vi "Target aquisition.vi"(8 "Ring Light Color":T2={"Hue"={119.53551591960586, 182.50767725024022}, "Sat"={103.21428571428572, 255.0}, "Val"={133.57142857142858, 255.0}} {"Hue" scale=0.0..255.0 scale format="%#_3g"}, 11 "Image":T3) -> (0 "Target tracking data":T1, 3 "Threshold image":T3, 4 "is there a target":bool)   [LabVIEW 2014]
uses:
  <vilib>/vision/Image Controls.llb/IMAQ Image.ctl
  <vilib>/vision/NI_Vision_Development_Module.lvlib
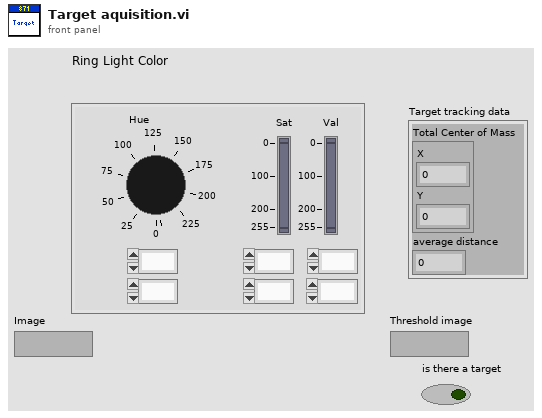
[diagram p1: front panel]
types:
  T1 = cluster{"Total Center of Mass":cluster{"X":dbl, "Y":dbl}, "average distance":dbl}
  T2 = cluster{"Hue":cluster{dbl, dbl}, "Sat":cluster{dbl, dbl}, "Val":cluster{dbl, dbl}}
  T3 = typedef "IMAQ Image.ctl" = refnum<image>
  T4 = cluster{"Area":dbl, "Number of Holes":dbl, "Bounding Rect":cluster{"Left":dbl, "Top":dbl, "Right":dbl, "Bottom":dbl}, "Center of Mass":cluster{"X":dbl, "Y":dbl}, "Orientation":dbl, "Dimensions":cluster{"Width":dbl, "Height":dbl}}[]
  T5 = typedef "target type.ctl" = cluster{"Area":dbl, "Number of Holes":dbl, "Bounding Rect":cluster{"Left":dbl, "Top":dbl, "Right":dbl, "Bottom":dbl}, "Center of Mass":cluster{"X":dbl, "Y":dbl}, "Orientation":dbl, "Dimensions":cluster{"Width":dbl, "Height":dbl}, "Shape Score X":dbl, "Aspect Ratio Score":dbl, "Area % Score":dbl, "Shape Score Y":dbl, "Am I Right?":bool, "distance":dbl}
  T6 = cluster{"Left Target":T5, "Right Target":T5, "Total Bounding Rect":cluster{"Left":dbl, "Top":dbl, "Right":dbl, "Bottom":dbl}, "Total Center of Mass":cluster{"X":dbl, "Y":dbl}}[]
  T7 = cluster{"Left Target":T5, "Right Target":T5, "Total Bounding Rect":cluster{"Left":dbl, "Top":dbl, "Right":dbl, "Bottom":dbl}, "Total Center of Mass":cluster{"X":dbl, "Y":dbl}}
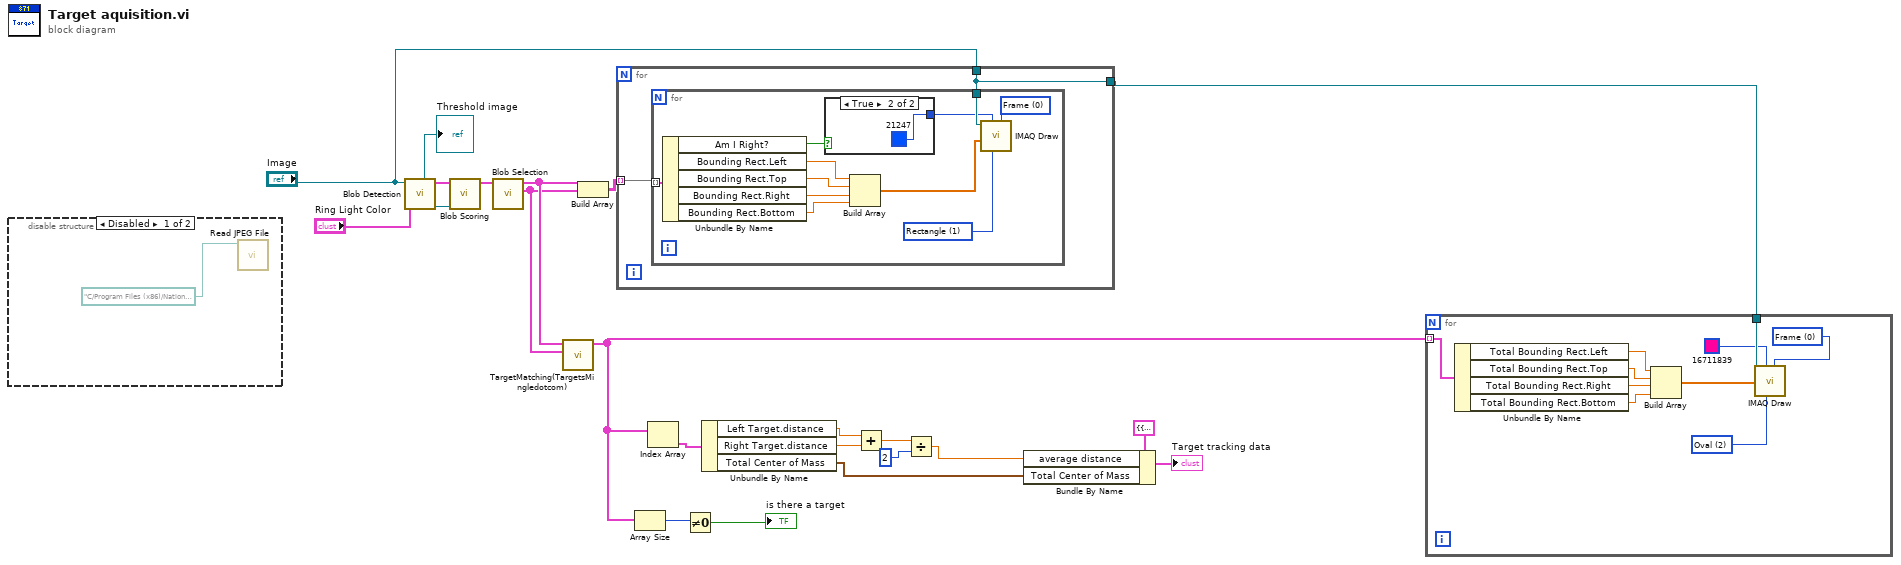
[diagram p0: block diagram]
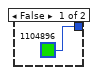
[diagram p2: hidden frame]
diagram:
  n1 = disable-structure shown="Disabled" {
    frame Disabled {
      n2 = call <vilib>:"Read JPEG File.vi"("path to JPEG file"=path "C:/Program Files (x86)/National Instruments/LabVIEW 2014/examples/FRC/roboRIO/Vision/2015 Vision Example/Sample Images/image.jpg") -> ()  [unwired: 8 in, 3 out]
    }
    frame Enabled {
    }
  }
  n3 = call "Blob Detection.vi"("Ring Light Color"="Ring Light Color", "Image"="Image") -> ("HSL Image"=w22:T3, "Acceptable Blobs"=w21:T4, "Image 2"=→"Threshold image":T3)  [unwired: 6 in]
  n4 = call "Blob Scoring.vi"("HSL Image"=w22, "Acceptable Blobs"=w21) -> ("Acceptable Blobs + Scores"=w19:T5[])  [unwired: 9 in]
  n5 = call "Blob Selection.vi"("Acceptable Blobs + Scores"=w19) -> ("Acceptable Left Blobs"=w15:T5[], "Acceptable Right Blobs"=w16:T5[])  [unwired: 9 in]
  n6 = call "TargetMatching(TargetsMingledotcom).vi"("Left Targets"=w15, "Right Targets"=w16) -> ("Target Set"=w11:T6)  [unwired: 9 in]
  n7 = Build Array(w16, w15) -> (w17:T5[][])
  n8 = for {
    tunnel: "Image" -> [w24]
    tunnel: w17 -> [w25] mode=indexing
    tunnel: [w24] -> w13
    n9 = for {
      tunnel: w25 -> [w36] mode=indexing
      tunnel: w24 -> [w34]
      w26 = u16 1 items=["Line", "Rectangle", "Oval"] ("Shape to draw")
      w32 = u16 0 items=["Frame", "Paint", "Invert Frame", "Invert Paint"] ("Draw Mode")
      n10 = Unbundle By Name(w36) -> ("Am I Right?"=w35:bool, "Bounding Rect.Left"=w31:dbl, "Bounding Rect.Top"=w30:dbl, "Bounding Rect.Right"=w29:dbl, "Bounding Rect.Bottom"=w28:dbl)
      n11 = case shown="True" w35 {
        tunnel: [u32 1104896 ("Color Box") u32 21247 ("Color Box")] -> w33
        frame False {
        }
        frame True {
        }
      }
      n12 = Build Array(w31, w30, w29, w28) -> (w27:dbl[])
      n13 = call "IMAQ Draw"("Draw Mode"=w32, "Shape to draw"=w26, "Pixel Color"=w33, "Coordinates"=w27, "Image Src"=w34) -> ()  [unwired: 5 in, 2 out]
    }
  }
  n14 = Array Size(array=w11) -> (size(s)=w2:i32)
  n15 = Index Array(array=w11) -> (element=w12:T7)  [unwired: 1 in]
  n16 = Not Equal To 0?(x=w2) -> (x != 0?=→"is there a target":bool)
  n17 = Unbundle By Name(w12) -> ("Left Target.distance"=w8:dbl, "Right Target.distance"=w3:dbl, "Total Center of Mass"=w4:cluster{"X":dbl, "Y":dbl})
  n18 = Add(x=w8, y=w3) -> (x+y=w6:dbl)
  n19 = Divide(x=w6, y=2) -> (x/y=w5:dbl)
  n20 = Bundle By Name(cluster=T1 {"Total Center of Mass"={"X"=0.0, "Y"=0.0}, "average distance"=0.0} ("Target tracking data"), "average distance"=w5, "Total Center of Mass"=w4) -> (→"Target tracking data":T1)
  n21 = for {
    tunnel: w11 -> [w48] mode=indexing
    tunnel: w13 -> [w42]
    w39 = u16 2 items=["Line", "Rectangle", "Oval"] ("Shape to draw")
    w40 = u16 0 items=["Frame", "Paint", "Invert Frame", "Invert Paint"] ("Draw Mode")
    n22 = Unbundle By Name(w48) -> ("Total Bounding Rect.Left"=w47:dbl, "Total Bounding Rect.Top"=w46:dbl, "Total Bounding Rect.Right"=w45:dbl, "Total Bounding Rect.Bottom"=w44:dbl)
    n23 = Build Array(w47, w46, w45, w44) -> (w43:dbl[])
    n24 = call "IMAQ Draw"("Draw Mode"=w40, "Shape to draw"=w39, "Pixel Color"=u32 16711839 ("Color Box"), "Coordinates"=w43, "Image Src"=w42) -> ()  [unwired: 5 in, 2 out]
  }
